vi "resample 200Hz.vi"(10 "Original Waveforms":waveform(sgl)[](array[waveform]), 11 "SamplingInfo":T1={"Number of Channels"=4, "Sampling Rate"=4.0, "Channels"=[], "Units"=[], "Offsets"=[]}) -> (2 "Resampled Waveforms":waveform(sgl)[](array[waveform]))   [LabVIEW 2017, in "TSNcDAQ_AI.lvlib"]
uses:
  <vilib>/addons/InsightCM/Devices/Shared/Cms/DAQmx/TSNcDAQ_AI.lvlib
  <vilib>/addons/InsightCM/Devices/Shared/Cms/cRIOWfmAcq/subVIs/RIO Wfm Cust Ctrls/rwfm_SamplingInfo.ctl
  <vilib>/measure/maresamp.llb/Resample Waveform (single shot).vi
  <vilib>/measure/NI_MAPro.lvlib
  <vilib>/addons/InsightCM/Devices/Shared/Cms/cRIOWfmAcq/cRIOWfmLib.lvlib
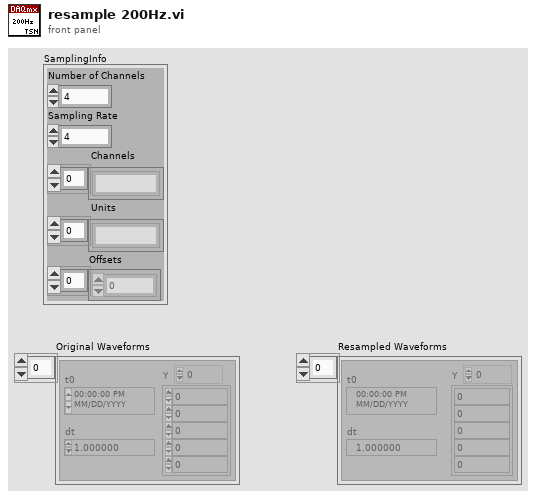
[diagram p1: front panel]
types:
  T1 = typedef "cRIOWfmLib.lvlib/rwfm_SamplingInfo.ctl" = cluster{"Number of Channels":i32, "Sampling Rate":dbl, "Channels":string[], "Units":string[], "Offsets":sgl[]}
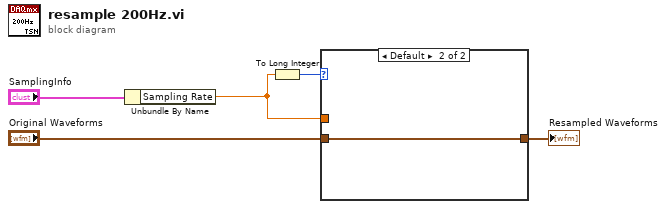
[diagram p0: block diagram]
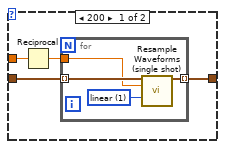
[diagram p2: hidden frame]
diagram:
  n1 = Unbundle By Name("SamplingInfo") -> ("Sampling Rate"=w2:dbl)
  n2 = To Long Integer(number=w2) -> (32bit integer=w1:i32)
  n3 = case shown="Default" w1 {
    tunnel: "Original Waveforms" -> [w9 w14]
    tunnel: [w6 w14] -> w3
    tunnel: w2 -> [w8 _]
    frame 200 {
      n4 = Reciprocal(x=w8) -> (1/x=w7:dbl)
      n5 = for {
        tunnel: w9 -> [w13] mode=indexing
        tunnel: w7 -> [w11]
        tunnel: [w12] -> w6 mode=indexing
        w10 = u16 1 items=["coerce", "linear", "spline", "FIR filter"] ("interpolation mode")
        n6 = call-poly <vilib>:"Resample Waveforms (single shot).vi"("waveform in"=w13, "dt"=w11, "interpolation mode"=w10) -> ("resampled waveform out"=w12:waveform(dbl))  [unwired: 9 in, 3 out]
      }
    }
    frame Default {
    }
  }
  "Resampled Waveforms" <- w3
